vi "calcDemandedSteps.vi"(8 "error in (no error)":errorcluster, 9 "loopPeriod":dbl[unit]=5000.0 min=10.0 max=5000.0, 10 "step rate limit (mag)":dbl[unit]=5000000.0 min=10000.0 max=5000000.0, 11 "SystemController in":refnum<class "SystemController.lvclass">) -> (0 "error out":errorcluster, 2 "step demand":dbl=5000.0 min=10.0 max=5000.0, 3 "SystemController out":refnum<class "SystemController.lvclass">)   [LabVIEW 2013, in "SystemController.lvclass"]
uses:
  SystemController.lvclass
  SystemController.lvclass/SystemController.ctl
  <vilib>/addons/control/pid/NI_PID_pid.lvlib
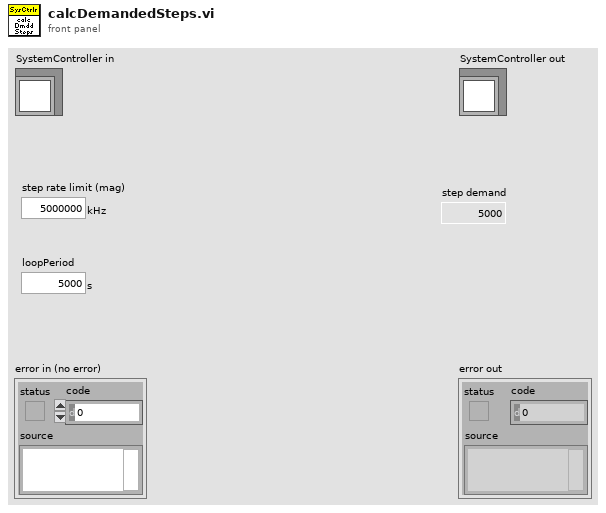
[diagram p1: front panel]
types:
  T1 = cluster{"proportional gain (Kc)":dbl, "integral time (Ti, min)":dbl, "derivative time (Td, min)":dbl}
  T2 = typedef "M2AADTTypedefs.lvlib/ForceDemand.ctl" = dbl[unit]
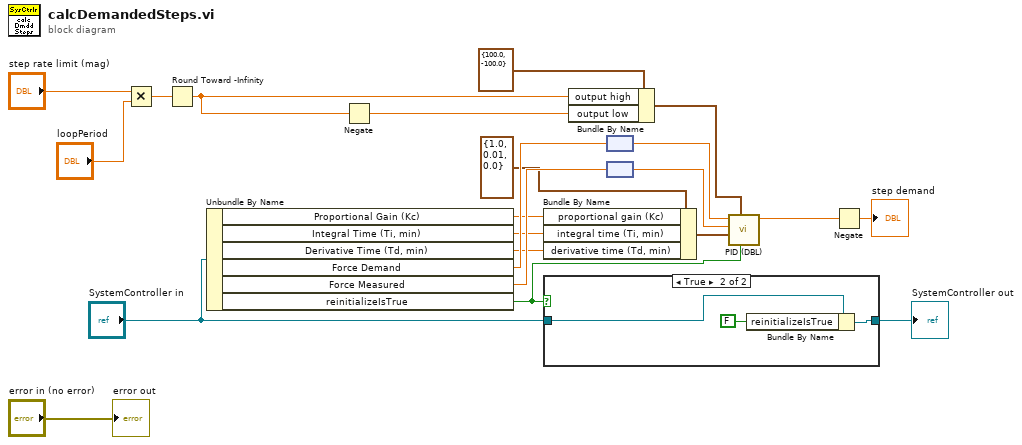
[diagram p0: block diagram]
diagram:
  n1 = Multiply(x="step rate limit (mag)", y="loopPeriod") -> (x*y=w16:dbl)
  n2 = Round Toward -Infinity(1:w16) -> (0:w1:dbl)
  n3 = Unbundle By Name("SystemController in") -> ("Proportional Gain (Kc)"=w11:dbl, "Integral Time (Ti, min)"=w10:dbl, "Derivative Time (Td, min)"=w8:dbl, "Force Demand"=w20:T2, "Force Measured"=w19:T2, "reinitializeIsTrue"=w5:bool)
  n4 = Negate(x=w1) -> (-x=w15:dbl)
  n5 = Bundle By Name(cluster=T1 {"proportional gain (Kc)"=1.0, "integral time (Ti, min)"=0.01, "derivative time (Td, min)"=0.0} ("PID gains"), "proportional gain (Kc)"=w11, "integral time (Ti, min)"=w10, "derivative time (Td, min)"=w8) -> (w9:T1)
  n6 = case shown="True" w5 {
    tunnel: [w23 w25] -> w7
    tunnel: "SystemController in" -> [w23 w26]
    frame False {
    }
    frame True {
      n7 = Bundle By Name(cluster=w26, "reinitializeIsTrue"=FALSE ("reinitialize? (F)")) -> (w25:refnum<class "SystemController.lvclass">)
    }
  }
  "SystemController out" <- w7
  n8 = Bundle By Name(cluster=cluster{"output high":dbl, "output low":dbl} {"output high"=100.0, "output low"=-100.0} ("output range"), "output high"=w1, "output low"=w15) -> (w14:cluster{"output high":dbl, "output low":dbl})
  n9 = node(w20) -> (w4:dbl)
  n10 = node(w19) -> (w3:dbl)
  n11 = call <vilib>:"PID (DBL).vi"("reinitialize? (F)"=w5, "output range"=w14, "PID gains"=w9, "process variable"=w3, "setpoint"=w4) -> ("output"=w13:dbl)  [unwired: 5 in, 1 out]
  n12 = Negate(x=w13) -> (-x=→"step demand":dbl)
  "error out" <- "error in (no error)"
